vi "KVMap-Merge.vi"(9 "Cluster 2":cluster{string[], string[]}, 10 "Cluster in":cluster{string[], string[]}) -> (3 "Cluster":cluster{string[], string[]})   [LabVIEW 2017]
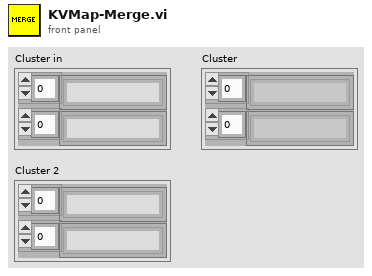
[diagram p1: front panel]
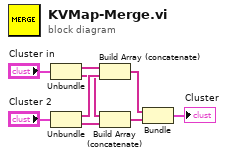
[diagram p0: block diagram]
diagram:
  n1 = Unbundle("Cluster in") -> (w3:string[], w4:string[])
  n2 = Unbundle("Cluster 2") -> (w5:string[], w6:string[])
  n3 = Build Array (concatenate)(w3, w5) -> (w7:string[])
  n4 = Build Array (concatenate)(w4, w6) -> (w8:string[])
  n5 = Bundle(w7, w8) -> (→"Cluster":cluster{string[], string[]})  [unwired: 1 in]
